vi "GetClassTemplates.vi"(0 "ClassWriter in":refnum<class "ClassWriter.lvclass">, 1 "DerivedFromThisClass(if any)":refnum<vi>, 5 "error in (no error)":errorcluster) -> (14 "ClassWriter out":refnum<class "ClassWriter.lvclass">, 15 "Templates":T1[](array[typedef]), 19 "error out":errorcluster)   [LabVIEW 2020, in "ClassWriter.lvclass"]
uses:
  ClassWriter.lvclass
  ClassTemplateType.ctl
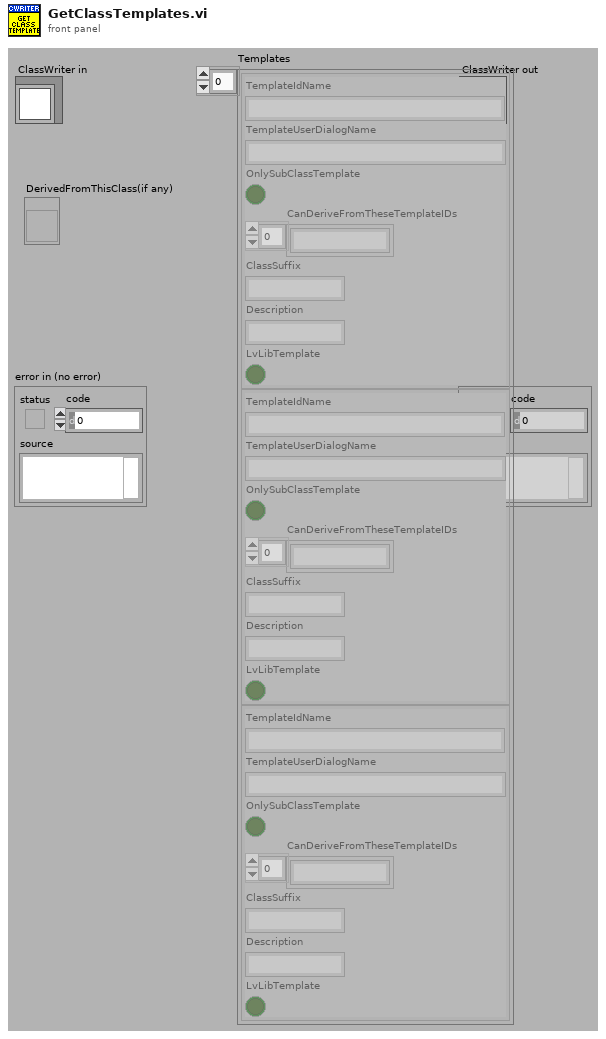
[diagram p1: front panel]
types:
  T1 = typedef "ClassWriter.lvclass/ClassTemplateType.ctl" = cluster{"TemplateIdName":string, "TemplateUserDialogName":string, "OnlySubClassTemplate":bool, "CanDeriveFromTheseTemplateIDs":string[], "ClassSuffix":string, "Description":string, "LvLibTemplate":bool}
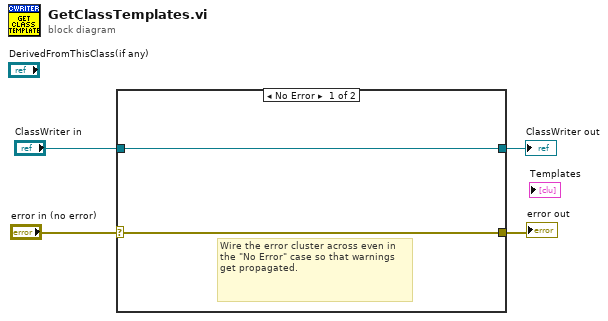
[diagram p0: block diagram]
diagram:
  n1 = case shown="No Error" "error in (no error)" {
    selector: "error in (no error)" -> [w5 w8]
    tunnel: [w5 w8] -> w3
    tunnel: [w6 w7] -> w1
    tunnel: "ClassWriter in" -> [w6 w7]
    frame No Error {
      # "Wire the error cluster across even in the \"No Error\" case so that warnings get propagated."
    }
    frame Error {
    }
  }
  "error out" <- w3
  "ClassWriter out" <- w1
